vi "dosimat876_fill.vi"(2 "error in":errorcluster, 3 "Dosimat Port In":refnum<visa-resource-name>="COM1") -> (0 "error out":errorcluster, 1 "Dosimat Port Out":refnum<visa-resource-name>="COM1")   [LabVIEW 2010]
panel:
  # "mooseNote: tell the Dosimat to fill... before this gets called\nthe vent relay (4) needs to be opened. And then\nclosed afterwards."
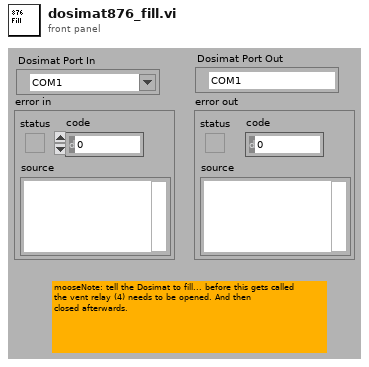
[diagram p1: front panel]
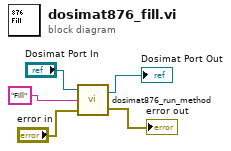
[diagram p0: block diagram]
diagram:
  n1 = call "dosimat876_run_method.vi"("error in"="error in", "Method"="Fill", "Dosimat Port In"="Dosimat Port In") -> ("error out"=→"error out":errorcluster, "Dosimat Port Out"=→"Dosimat Port Out":refnum<visa-resource-name>)
